vi "Notify Monitor.vi"(8 "error in (no error)":errorcluster, 11 "Monitored Actor in":refnum<class "Monitored Actor.lvclass">) -> (0 "error out":errorcluster, 3 "Monitored Actor out":refnum<class "Monitored Actor.lvclass">)   [LabVIEW 2018, in "Monitored Actor.lvlib" / "Monitored Actor.lvclass"]
doc: "Sends a message the the actor monitor that a new actor has been spawned. Supplies it with the appropriate data so the monitor can keep track of everything\n\nThis VI cannot be called from pre-launch init. It must be called from a Do method. This is because it may need to launch a new instance of the actor monitor window.\n\nCopyright: MGI\nAuthored by: Derek Trepanier"
uses:
  Monitored Actor.lvclass
  C:/Program Files (x86)/National Instruments/LabVIEW 2018/vi.lib/ActorFramework/Actor/Actor.lvclass
  <vilib>/ActorFramework/Actor/Actor.lvclass/Actor.ctl
  <vilib>/ActorFramework/Message Enqueuer/Message Enqueuer.lvclass/Message Enqueuer.ctl
  Monitored Actor.lvclass/Monitored Actor.ctl
  Actor Monitor/Actor Monitor Messages/Actor Launched Msg/Actor Launched Msg.lvclass/Actor Launched Msg.ctl
  <vilib>/ActorFramework/Message Enqueuer/Init from Existing Queue.vi
  <vilib>/ActorFramework/Message Enqueuer/Enqueue.vi
  Actor Monitor/Actor Monitor Messages/Actor Launched Msg/Actor Launched Msg.lvclass
  C:/Program Files (x86)/National Instruments/LabVIEW 2018/vi.lib/ActorFramework/Message/Message.lvclass
  <vilib>/ActorFramework/Message Priority Queue/Priority Enqueue.vi
  <vilib>/ActorFramework/Message Enqueuer/Message Enqueuer.lvclass
  <vilib>/ActorFramework/Actor/Actor.lvclass
  Actor Monitor/Actor/Actor Monitor.lvclass
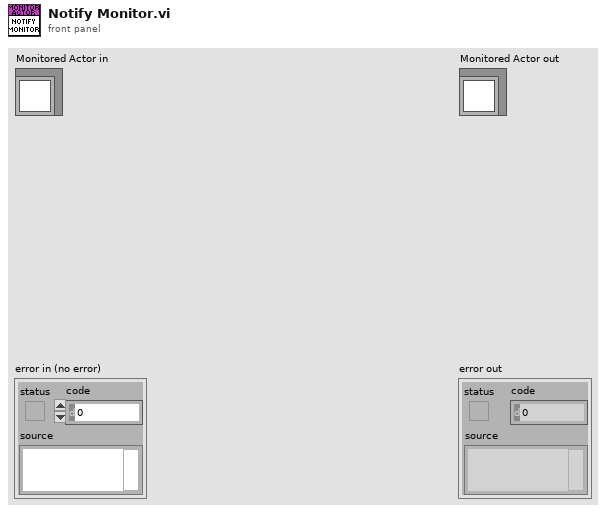
[diagram p1: front panel]
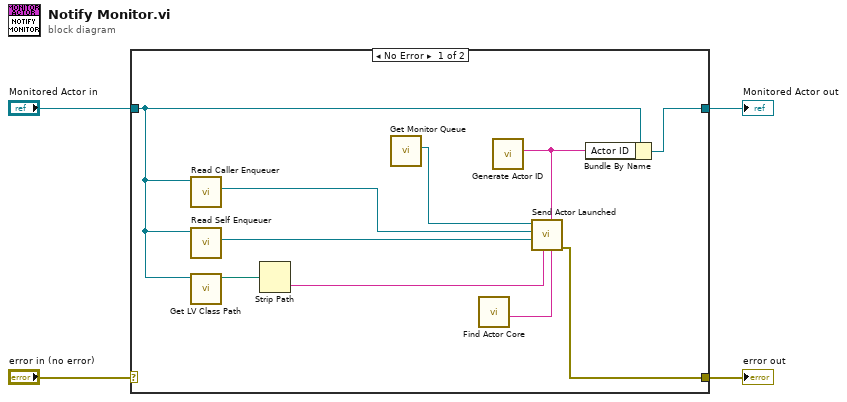
[diagram p0: block diagram]
diagram:
  n1 = case shown="No Error" "error in (no error)" {
    selector: "error in (no error)" -> [_ w16]
    tunnel: [w6 w16] -> w1
    tunnel: [w7 w15] -> w2
    tunnel: "Monitored Actor in" -> [w13 w15]
    frame No Error {
      n2 = call <vilib>:"Read Caller Enqueuer.vi"("Actor"=w13) -> ("Caller Enqueuer"=w11:refnum<class "Message Enqueuer.lvclass">)  [unwired: 10 in]
      n3 = call <vilib>:"Read Self Enqueuer.vi"("Actor"=w13) -> ("Self Enqueuer"=w12:refnum<class "Message Enqueuer.lvclass">)  [unwired: 10 in]
      n4 = call <vilib>:"Get LV Class Path.vi"("object"=w13) -> ("class path"=w14:path)  [unwired: 9 in, 1 out]
      n5 = Strip Path(path=w14) -> (name=w10:string)  [unwired: 1 out]
      n6 = call "Get Monitor Queue.vi"() -> ("Caller Enqueuer"=w8:refnum<class "Message Enqueuer.lvclass">)  [unwired: 11 in]
      n7 = call "Find Actor Core.vi"() -> ("Actor Core VI Name"=w5:string)  [unwired: 10 in, 1 out]
      n8 = call "Generate Actor ID.vi"() -> ("Actor ID"=w9:string)  [unwired: 11 in]
      n9 = call "Send Actor Launched.vi"("Actor Core Name"=w5, "Actor ID"=w9, "Class Name"=w10, "Actor's Queue"=w12, "Actor's Caller"=w11, "Message Enqueuer"=w8) -> ("error out"=w6:errorcluster)  [unwired: 4 in, 1 out]
      n10 = Bundle By Name(cluster=w13, "Actor ID"=w9) -> (w7:refnum<class "Monitored Actor.lvclass">)
    }
    frame Error {
    }
  }
  "error out" <- w1
  "Monitored Actor out" <- w2
